vi "Measurement Logic.vi"() -> ()   [LabVIEW 2021, in "Crosstalk_Audio DAC.lvlib"]
uses:
  Crosstalk_Audio DAC.lvlib
  <vilib>/PDM Acquisition Toolkit/host/Classes/Channels/I2S Ouput/Controls/GenerationChannelProperties.ctl
  <vilib>/PDM Acquisition Toolkit/host/Classes/Channels/I2S Ouput/I2S Output Channel.lvclass
  <vilib>/PDM Acquisition Toolkit/host/Classes/Tasks/I2S Output/Control/SignalProperties.ctl
  <vilib>/PDM Acquisition Toolkit/host/Classes/Tasks/I2S Output/I2S Output Task.lvclass
  shared/controls/Digital Initialize Settings.ctl
  shared/digital audio protocol/digital audio protocol controls.lvlib
  shared/controls/Single Tone Measurement Settings.ctl
  shared/controls/Single Tone Filter Settings.ctl
  shared/controls/Analog Initialize Settings.ctl
  Measurement Configuration.ctl
  Measurement Results.ctl
  <vilib>/Plug-In SDKs/Measurements/Measure Call Context/Measure Call Context.lvclass
panel:
  out "measure call context out":refnum<class "Measure Call Context.lvclass">
  in  "measure call context in":refnum<class "Measure Call Context.lvclass">
  out "measurement results":T1 {"Crosstalks" format="%_6g"; "Frequencies" format="%_6g"; "df" format="%_6g"; "f0" format="%_6g"; "dt" format="%_6g"; "Frequency domain" format="%_6g"; "Time domain" format="%_6g"}
  in  "measurement configuration":T2={"Frequency (Hz)"=1000.0, "Protocol file"="", "Digital audio channel"="", "Master clock channel"="", "Output level"=0.0, "Output level units"="dBFS", "Output range (Vpk-pk)"=5.74, "Victim channel"="", "Interferrer channel"="", "Sample rate (Hz)"=51200.0, "Min measurement cycles"=0, "Min measurement time (s)"=0.1, "Min settling cycles"=0, "Min settling time (s)"=0.1, "Highpass filter"="AC", "Lowpass filter"="AES17_20kHz", "Weighting filter"="A-weighting", "Band start (Hz)"=20.0, "Band stop (Hz)"=20000.0, "Interferrer channel number"=20000} {"Band stop (Hz)" format="%#_6pHz"; "Band start (Hz)" format="%#_6pHz"; "Min settling time (s)" format="%#_6ps"; "Min measurement time (s)" format="%#_6ps"; "Sample rate (Hz)" format="%#_6pHz"; "Output range (Vpk-pk)" format="%.3p Vpk-pk"; "Output level" format="%#_6p"; "Frequency (Hz)" format="%#_6pHz"}
  out "error out":errorcluster
  in  "error in":errorcluster
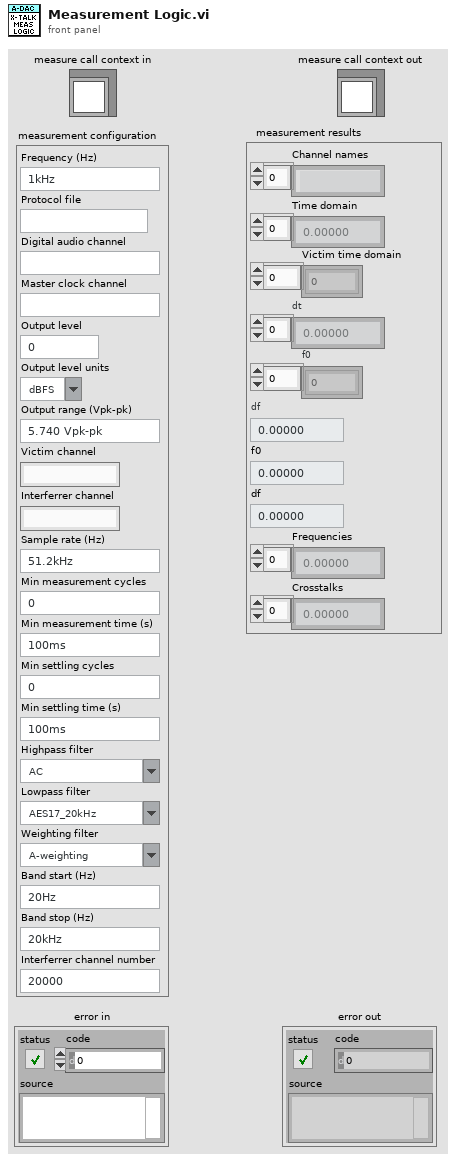
[diagram p1: front panel]
types:
  T1 = typedef "Crosstalk_Audio DAC.lvlib/Measurement Results.ctl" = cluster{"Channel names":string[], "Time domain":dbl[], "Victim time domain":dbl[], "Frequency domain":dbl[], "Victim frequency domain":dbl[], "dt":dbl, "f0":dbl, "df":dbl, "Frequencies":dbl[], "Crosstalks":dbl[]}
  T2 = typedef "Crosstalk_Audio DAC.lvlib/Measurement Configuration.ctl" = cluster{"Frequency (Hz)":dbl, "Protocol file":string, "Digital audio channel":string, "Master clock channel":string, "Output level":dbl, "Output level units":string, "Output range (Vpk-pk)":dbl, "Victim channel":string, "Interferrer channel":string, "Sample rate (Hz)":dbl, "Min measurement cycles":u32, "Min measurement time (s)":dbl, "Min settling cycles":u32, "Min settling time (s)":dbl, "Highpass filter":string, "Lowpass filter":string, "Weighting filter":string, "Band start (Hz)":dbl, "Band stop (Hz)":dbl, "Interferrer channel number":i32}
  T3 = typedef "Analog Initialize Settings.ctl" = cluster{"analog acquisition channel":string, "samples per channel":i32, "sample rate":dbl}
  T4 = typedef "Single Tone Filter Settings.ctl" = cluster{"Highpass filter":string, "Lowpass filter":string, "Weighting filter":string}
  T5 = typedef "Single Tone Measurement Settings.ctl" = cluster{"Band start":dbl, "Band stop":dbl, "Amplitude":dbl, "Frequency":dbl, "Full scale range":dbl}
  T6 = typedef "Digital Initialize Settings.ctl" = cluster{"digital channel list":string, "master clock channel list":string, "protocol settings file path":path, "signal parameters":T7}
  T7 = typedef "PDM Acquisition Class Library.lvlib/I2S Output Task.lvclass/SignalProperties.ctl" = cluster{"cyclic signal":dbl[], "channel parameters":T8[]}
  T8 = typedef "PDM Acquisition Class Library.lvlib/I2S Output Channel.lvclass/GenerationChannelProperties.ctl" = cluster{"cyclic period":dbl, "cyclic phase offset":dbl, "gain":dbl}
  T9 = typedef "digital audio protocol controls.lvlib/digital audio protocol settings.ctl" = cluster{"number of channels":u32, "data justification":string, "endianness":string, "channel length":u32, "bit depth":u32, "frame clock rate":dbl, "bit clock edge sync":string, "master clock rate":dbl, "logic level":string, "frame sync edge for channel 0":string, "Channel 0 Offset":u32}
  T10 = typedef "PDM Acquisition Class Library.lvlib/PCM Output Task.lvclass/PCM Output Task DVR.ctl" = refnum<data-value>
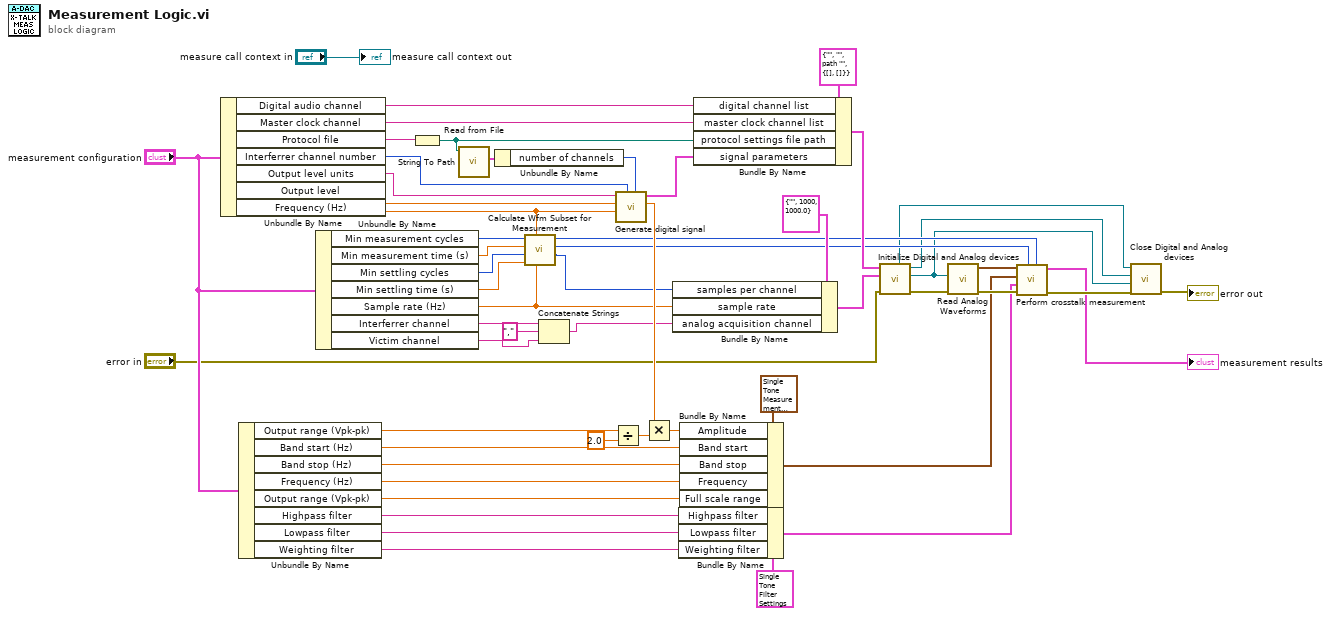
[diagram p0: block diagram]
diagram:
  n1 = Unbundle By Name("measurement configuration") -> ("Digital audio channel"=w52:string, "Master clock channel"=w53:string, "Protocol file"=w54:string, "Interferrer channel number"=w1:i32, "Output level units"=w48:string, "Output level"=w47:dbl, "Frequency (Hz)"=w7:dbl)
  n2 = Unbundle By Name("measurement configuration") -> ("Output range (Vpk-pk)"=w39:dbl, "Band start (Hz)"=w43:dbl, "Band stop (Hz)"=w42:dbl, "Frequency (Hz)"=w41:dbl, "Output range (Vpk-pk)"=w40:dbl, "Highpass filter"=w34:string, "Lowpass filter"=w33:string, "Weighting filter"=w32:string)
  n3 = Unbundle By Name("measurement configuration") -> ("Min measurement cycles"=w28:u32, "Min measurement time (s)"=w27:dbl, "Min settling cycles"=w26:u32, "Min settling time (s)"=w25:dbl, "Sample rate (Hz)"=w24:dbl, "Interferrer channel"=w10:string, "Victim channel"=w9:string)
  n4 = String To Path(string=w54) -> (path=w50:path)
  n5 = call "Read from File.vi"("file path"=w50) -> ("digital audio protocol settings"=w49:T9)  [unwired: 8 in, 2 out]
  n6 = Unbundle By Name(w49) -> ("number of channels"=w46:u32)
  n7 = call "Calculate Wfm Subset for Measurement.vi"("sampling rate"=w24, "signal frequency"=w7, "minimum settling duration"=w25, "minimum settling cycles"=w26, "minimum measurement duration"=w27, "minimum measurement cycles"=w28) -> ("total acquisition (samples)"=w23:u32, "duration (samples)"=w19:u32, "start (samples)"=w18:u32)  [unwired: 3 in]
  n8 = Concatenate Strings(w10, "," ("string"), w9) -> (w8:string)
  n9 = Divide(x=w39, y=2.0) -> (x/y=w37:dbl)
  n10 = call "Generate digital signal.vi"("number of channels"=w46, "interferrer channel"=w1, "frequency"=w7, "Output level in"=w47, "Output level units"=w48) -> ("Output level out"=w31:dbl, "Signal Properties"=w45:T7)  [unwired: 5 in]
  n11 = Multiply(x=w31, y=w37) -> (x*y=w36:dbl)
  n12 = Bundle By Name(cluster=T3 {"analog acquisition channel"="", "samples per channel"=1000, "sample rate"=1000.0} ("Analog initialize settings"), "samples per channel"=w23, "sample rate"=w24, "analog acquisition channel"=w8) -> (w20:T3)
  n13 = Bundle By Name(cluster=T4 {"Highpass filter"="DC", "Lowpass filter"="No filter", "Weighting filter"="A-weighting"} ("filter settings"), "Highpass filter"=w34, "Lowpass filter"=w33, "Weighting filter"=w32) -> (w5:T4)
  n14 = Bundle By Name(cluster=T5 {"Band start"=20.0, "Band stop"=20000.0, "Amplitude"=1.0, "Frequency"=1000.0, "Full scale range"=3.16} ("measurement settings"), "Amplitude"=w36, "Band start"=w43, "Band stop"=w42, "Frequency"=w41, "Full scale range"=w40) -> (w6:T5)
  n15 = Bundle By Name(cluster=T6 {"digital channel list"="", "master clock channel list"="", "protocol settings file path"=path "", "signal parameters"={"cyclic signal"=[], "channel parameters"=[]}} ("Digital initialize settings"), "digital channel list"=w52, "master clock channel list"=w53, "protocol settings file path"=w50, "signal parameters"=w45) -> (w29:T6)
  n16 = call "Initialize Digital and Analog devices.vi"("error in"="error in", "Analog initialize settings"=w20, "Digital initialize settings"=w29) -> ("error out"=w14:errorcluster, "analog task"=w15:refnum<k21>, "master clock task"=w16:T10, "digital audio task"=w17:T10)  [unwired: 5 in]
  n17 = call "Read Analog Waveforms.vi"("error in"=w14, "analog task"=w15) -> ("error out"=w13:errorcluster, "waveforms"=w30:waveform(dbl)[])  [unwired: 7 in, 1 out]
  n18 = call "Perform crosstalk measurement.vi"("start samples/time"=w18, "duration"=w19, "error in"=w13, "filter settings"=w5, "measurement settings"=w6, "waveforms"=w30) -> ("error out"=w12:errorcluster, "output cluster"=→"measurement results":T1)  [unwired: 4 in]
  n19 = call "Close Digital and Analog devices.vi"("error in"=w12, "analog task"=w15, "master clock task"=w16, "digital audio task"=w17) -> ("error out"=→"error out":errorcluster)  [unwired: 7 in]
  "measure call context out" <- "measure call context in"
